vi "ULx Create Channel (CompI-Counter Input-Position-Angular Encoder).vi"(0 "task in":refnum<k24>, 1 "decoding type":i32(ring)=2 items=["X1", "X2", "X4"], 2 "pulses per revolution":i32=24, 3 "initial angle":dbl, 5 "counters":refnum<k21>, 9 "units":i32(ring) items=["Degrees", "Radians", "Ticks"], 11 "error in":errorcluster, 12 "z index mode":i32(ring) items=["Disabled"=0, "LatchCounter"=8, "ResetCounter"=32]) -> (4 "task out":refnum<k24>, 15 "error out":errorcluster)   [LabVIEW 2020]
doc: "Creates a channel(s) that uses an angular encoder to measure angular position."
uses:
  C:/Users/William/Documents/LV 2020 builds/LeaktestDAQ/Source-v33/ULx_LV.dll
  ULx_LV.dll
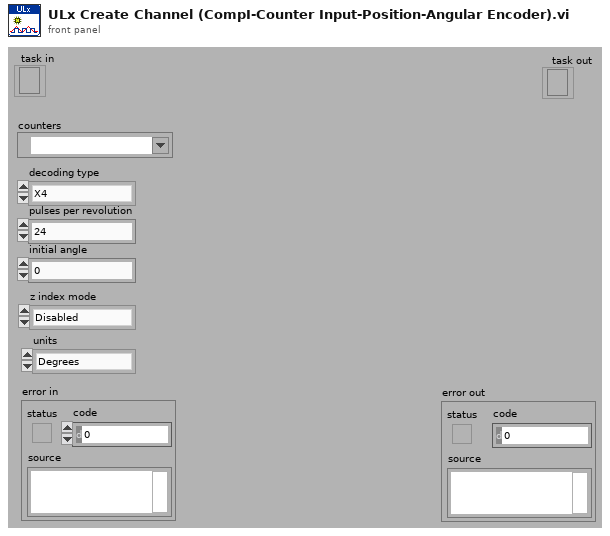
[diagram p1: front panel]
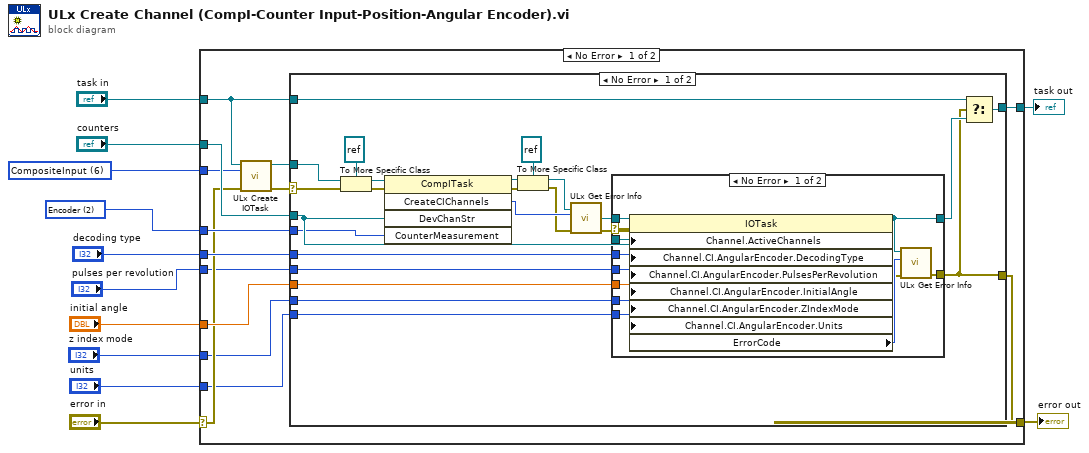
[diagram p0: block diagram]
diagram:
  w5 = 2 items=["CountEdges"=1, "Encoder"=2, "Frequency"=3, "Period"=4] ("CounterMeasurement")
  w8 = 6 items=["AnalogInput", "AnalogOutput", "DigitalInput", "DigitalOutput", "CounterInput", "CounterOutput", "CompositeInput", "CompositeOutput", "TemperatureInput"] ("taskType")
  n1 = case shown="No Error" "error in" {
    selector: "error in" -> [w17 w67]
    tunnel: "task in" -> [w13 w66]
    tunnel: "counters" -> [w22 _]
    tunnel: [w25 w66] -> w10
    tunnel: [w24 w67] -> w9
    tunnel: w8 -> [w21 _]
    tunnel: "decoding type" -> [w20 _]
    tunnel: "initial angle" -> [w19 _]
    tunnel: w5 -> [w18 _]
    tunnel: "pulses per revolution" -> [w16 _]
    tunnel: "z index mode" -> [w15 _]
    tunnel: "units" -> [w14 _]
    frame No Error {
      n2 = call "ULx Create IOTask.vi"("error in"=w17, "taskType"=w21, "i/o task in"=w13) -> ("error out"=w26:errorcluster, "i/o task out"=w23:refnum<k24>)  [unwired: 7 in]
      n3 = case shown="No Error" w26 {
        selector: w26 -> [w47 w65]
        tunnel: [w27 w65] -> w24
        tunnel: [w29 w64] -> w25
        tunnel: w23 -> [w45 _]
        tunnel: w22 -> [w42 _]
        tunnel: w20 -> [w39 _]
        tunnel: w19 -> [w41 _]
        tunnel: w18 -> [w40 _]
        tunnel: w16 -> [w38 _]
        tunnel: w15 -> [w37 _]
        tunnel: w14 -> [w36 _]
        tunnel: w13 -> [w30 w64]
        frame No Error {
          n4 = To More Specific Class(target class=refnum<k24> refnum, reference=w45, error in=w47) -> (specific class reference=w48:refnum<k24>, error out=w46:errorcluster)
          n5 = invoke class="CompITask" method="CreateCIChannels"(reference=w48, error in=w46, "DevChanStr"=w42, "CounterMeasurement"=w40) -> (reference out=w34:refnum<k24>, error out=w33:errorcluster, "CreateCIChannels"=w44:i32)  [unwired: 1 in, 2 out]
          n6 = To More Specific Class(target class=refnum<k24> refnum, reference=w34, error in=w33) -> (specific class reference=w31:refnum<k24>, error out=w32:errorcluster)
          n7 = call "ULx Get Error Info.vi"("error in"=w32, "ErrorCode"=w44, "task in"=w31) -> ("error out"=w43:errorcluster)  [unwired: 8 in]
          n8 = case shown="No Error" w43 {
            selector: w43 -> [w61 w63]
            tunnel: w31 -> [w60 w62]
            tunnel: w42 -> [w59 _]
            tunnel: [w56 w63] -> w27
            tunnel: w41 -> [w53 _]
            tunnel: w39 -> [w55 _]
            tunnel: w38 -> [w54 _]
            tunnel: w37 -> [w52 _]
            tunnel: w36 -> [w51 _]
            tunnel: [w50 w62] -> w28
            frame No Error {
              n9 = property class="IOTask"(reference=w60, error in=w61, "Channel.ActiveChannels"=w59, "Channel.CI.AngularEncoder.DecodingType"=w55, "Channel.CI.AngularEncoder.PulsesPerRevolution"=w54, "Channel.CI.AngularEncoder.InitialAngle"=w53, "Channel.CI.AngularEncoder.ZIndexMode"=w52, "Channel.CI.AngularEncoder.Units"=w51) -> (reference out=w50:refnum<k24>, error out=w57:errorcluster, "ErrorCode"=w58:i32)
              n10 = call "ULx Get Error Info.vi"("error in"=w57, "ErrorCode"=w58, "task in"=w50) -> ("error out"=w56:errorcluster)  [unwired: 8 in]
            }
            frame Error {
            }
          }
          n11 = Select(t=w30, s=w27, f=w28) -> (s? t:f=w29:refnum<k24>)
        }
        frame Error {
        }
      }
    }
    frame Error {
    }
  }
  "error out" <- w9
  "task out" <- w10
